vi "U8_To_U32.vi"(0 "U32 IN":u32, 7 "U8 IN":u8) -> (4 "U8 OUT":u8, 8 "U32 OUT":u32)   [LabVIEW 2016]
panel:
  # "Copyright (C) 2020 Edward S Allgeyer\n\nRedistribution and use in source and binary forms, with or without\nmodification, are permitted provided that the following conditions\nare met:\n\n1. Redistributions of source code must retain the above copyright\n   notice, this list of conditions and the following disclaimer.\n\n2. Redistributions in binary form must reproduce the above copyright\n   notice, this list of conditions and the following disclaimer in\n   the documentation and/or other materials provided with the\n   distribution.\n\n3. Neither the name of the copyright holder nor the names of its\n   contributors may be used to endorse or promote products derived\n   from this software without specific prior written permission.\n\nTHIS SOFTWARE IS PROVIDED BY THE COPYRIGHT HOLDERS AND CONTRIBUTORS\n\"AS IS\" AND ANY EXPRESS OR IMPLIED WARRANTIES, INCLUDING, BUT NOT\nLIMITED TO, THE IMPLIED WARRANTIES OF MERCHANTABILITY AND FITNESS\nFOR A PARTICULAR PURPOSE ARE DISCLAIMED. IN NO EVENT SHALL THE\nCOPYRIGHT HOLDER OR CONTRIBUTORS BE LIABLE FOR ANY DIRECT, INDIRECT,\nINCIDENTAL, SPECIAL, EXEMPLARY, OR CONSEQUENTIAL DAMAGES (INCLUDING,\nBUT NOT LIMITED TO, PROCUREMENT OF SUBSTITUTE GOODS OR SERVICES;\nLOSS OF USE, DATA, OR PROFITS; OR BUSINESS INTERRUPTION) HOWEVER\nCAUSED AND ON ANY THEORY OF LIABILITY, WHETHER IN CONTRACT, STRICT\nLIABILITY, OR TORT (INCLUDING NEGLIGENCE OR OTHERWISE) ARISING IN\nANY WAY OUT OF THE USE OF THIS SOFTWARE, EVEN IF ADVISED OF THE\nPOSSIBILITY OF SUCH DAMAGE."
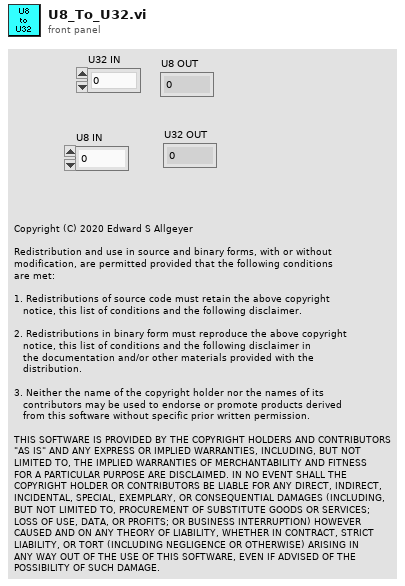
[diagram p1: front panel]
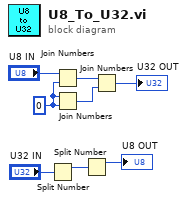
[diagram p0: block diagram]
diagram:
  w8 = u8 0
  n1 = Split Number(x="U32 IN") -> (hi(x)=w2:u16)  [unwired: 1 out]
  n2 = Join Numbers(hi="U8 IN", lo=w8) -> ((hi.lo)=w6:u16)
  n3 = Join Numbers(hi=w8, lo=w8) -> ((hi.lo)=w7:u16)
  n4 = Split Number(x=w2) -> (hi(x)=→"U8 OUT":u8)  [unwired: 1 out]
  n5 = Join Numbers(hi=w6, lo=w7) -> ((hi.lo)=→"U32 OUT":u32)
